vi "TBM.GetChangedControl.vi"(8 "error in (no error)":errorcluster, 10 "NewVal":variant, 11 "OldVal":variant) -> (0 "error out":errorcluster, 3 "Changed Control":cluster{"Data Name":string, "VElement":variant})   [LabVIEW 2013, in "ToolbarMenu.lvlib"]
uses:
  ToolbarMenu.lvlib
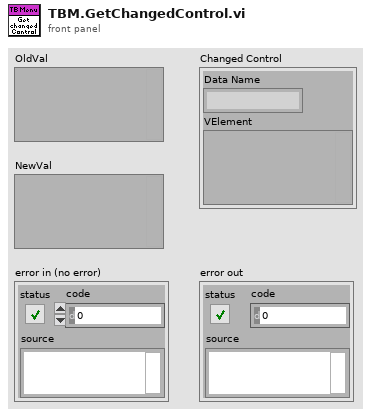
[diagram p1: front panel]
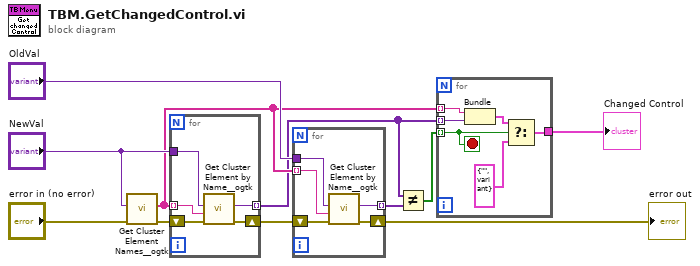
[diagram p0: block diagram]
diagram:
  n1 = call <userlib>:"Get Cluster Element Names__ogtk.vi"("error in (no error)"="error in (no error)", "Cluster"="NewVal") -> ("error out"=w5:errorcluster, "Element Names"=w7:string[])  [unwired: 8 in]
  n2 = for {
    tunnel: "NewVal" -> [w16]
    tunnel: w7 -> [w15] mode=indexing
    tunnel: [w14] -> w1 mode=indexing
    shift-right: [w13] -> w4
    shift-left: w5 -> [w12]
    n3 = call <userlib>:"Get Cluster Element by Name__ogtk.vi"("error in (no error)"=w12, "Element Name"=w15, "Cluster"=w16) -> ("error out"=w13:errorcluster, "VElement"=w14:variant)  [unwired: 6 in, 1 out]
  }
  n4 = for {
    tunnel: "OldVal" -> [w21]
    tunnel: w7 -> [w20] mode=indexing
    tunnel: [w19] -> w2 mode=indexing
    shift-right: [w18] -> w3
    shift-left: w4 -> [w17]
    n5 = call <userlib>:"Get Cluster Element by Name__ogtk.vi"("error in (no error)"=w17, "Element Name"=w20, "Cluster"=w21) -> ("error out"=w18:errorcluster, "VElement"=w19:variant)  [unwired: 6 in, 1 out]
  }
  "error out" <- w3
  n6 = Not Equal?(x=w1, y=w2) -> (x != y?=w6:bool[])
  n7 = for {
    tunnel: w6 -> [w26] mode=indexing
    tunnel: w1 -> [w24] mode=indexing
    tunnel: w7 -> [w27] mode=indexing
    tunnel: [w25] -> w8
    stop <- w26 stop-if-true
    n8 = Bundle("Data Name"=w27, "VElement"=w24) -> (w23:cluster{"Data Name":string, "VElement":variant})  [unwired: 1 in]
    n9 = Select(t=w23, s=w26, f=cluster{"Data Name":string, "VElement":variant} {"Data Name"="", "VElement"=variant}) -> (s? t:f=w25:cluster{"Data Name":string, "VElement":variant})
  }
  "Changed Control" <- w8
